vi "Enqueue Message.vi"(8 "Error in":errorcluster, 9 "Data":variant, 10 "Cmd":string, 11 "Queue Data":T1) -> (0 "Error out":errorcluster)   [LabVIEW 2018, in "Queue Messaging.lvlib"]
uses:
  Queue Messaging.lvlib
  QMH Template/Type Defs/EventsAndQueues--cluster.ctl
  Type Defs/Queue Message--cluster.ctl
  Event Messaging/Type Defs/Event Message--cluster.ctl
  QMH/QMH CORE.lvlib
  Event Messaging/Event Messaging.lvlib
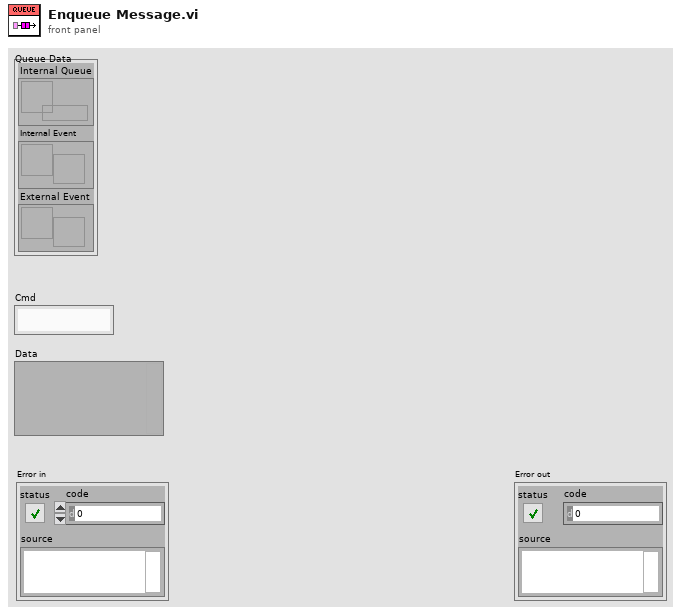
[diagram p1: front panel]
types:
  T1 = typedef "QMH CORE.lvlib/EventsAndQueues--cluster.ctl" = cluster{"Internal Queue":refnum<queue>, "Internal Event":refnum<user-event>, "External Event":refnum<user-event>}
  T2 = typedef "Queue Messaging.lvlib/Queue Message--cluster.ctl" = cluster{"Cmd":string, "Data":variant}
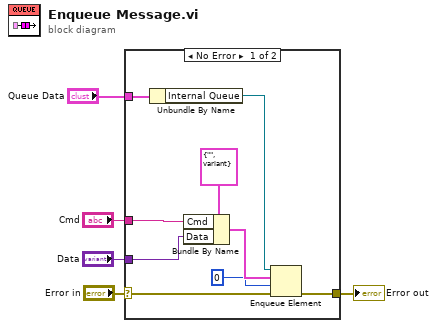
[diagram p0: block diagram]
diagram:
  n1 = case shown="No Error" "Error in" {
    selector: "Error in" -> [w12 w15]
    tunnel: [w11 w15] -> w4
    tunnel: "Cmd" -> [w10 _]
    tunnel: "Data" -> [w9 _]
    tunnel: "Queue Data" -> [w8 _]
    frame No Error {
      n2 = Unbundle By Name(w8) -> ("Internal Queue"=w7:refnum<queue>)
      n3 = Bundle By Name(cluster=T2 {"Cmd"="", "Data"=variant} ("Message"), "Cmd"=w10, "Data"=w9) -> (w13:T2)
      n4 = Enqueue Element(queue=w7, element=w13, timeout in ms (-1)=0, error in (no error)=w12) -> (error out=w11:errorcluster)  [unwired: 2 out]
    }
    frame Error {
    }
  }
  "Error out" <- w4
